vi "Get Description of Shared Variables.vi"(8 "error in":errorcluster, 11 "Variable References In":refnum<k21>[](array[refnum])) -> (0 "error out":errorcluster, 2 "Variable Descriptions":T1[](array[typedef]), 3 "Variable References Out":refnum<k21>[](array[refnum]))   [LabVIEW 2017, in "Shared Variables Library.lvlib"]
doc: "Retrieves the Name, URL and Datatype from an array of shared variable references."
uses:
  Shared Variables Library.lvlib
  Typedefs/Shared Variable Properties--Cluster.ctl
  <resource>/objmgr/ni.var.rc
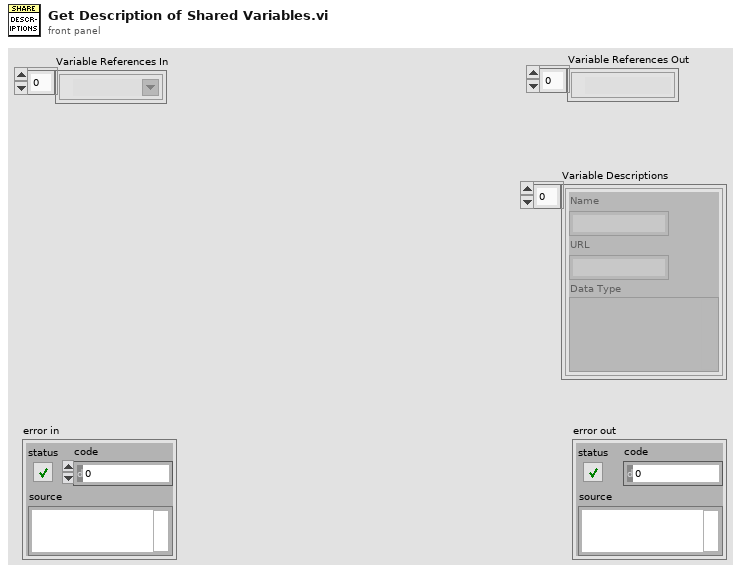
[diagram p1: front panel]
types:
  T1 = typedef "Shared Variables Library.lvlib/Shared Variable Properties--Cluster.ctl" = cluster{"Name":string, "URL":string, "Data Type":variant}
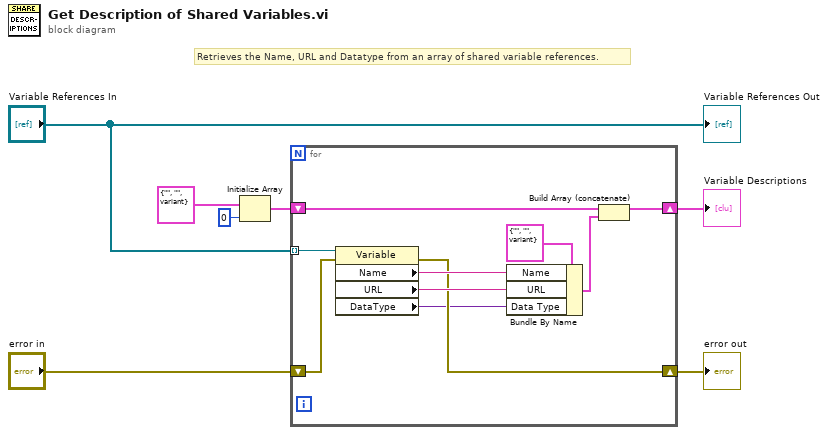
[diagram p0: block diagram]
diagram:
  # "Retrieves the Name, URL and Datatype from an array of shared variable references."
  n1 = Initialize Array(T1 {"Name"="", "URL"="", "Data Type"=variant} ("Shared Variable Data"), 0 ("dimension size")) -> (w4:T1[])
  n2 = for {
    tunnel: "Variable References In" -> [w17] mode=indexing
    shift-right: [w15] -> w5
    shift-left: w4 -> [w16]
    shift-right: [w11] -> w7
    shift-left: "error in" -> [w14]
    n3 = property class="Variable"(reference=w17, error in=w14) -> (error out=w11:errorcluster, "Name"=w13:string, "URL"=w12:string, "DataType"=w10:variant)  [unwired: 1 out]
    n4 = Bundle By Name(cluster=T1 {"Name"="", "URL"="", "Data Type"=variant} ("Shared Variable Data"), "Name"=w13, "URL"=w12, "Data Type"=w10) -> (w8:T1)
    n5 = Build Array (concatenate)(w16, w8) -> (w15:T1[])
  }
  "error out" <- w7
  "Variable Descriptions" <- w5
  "Variable References Out" <- "Variable References In"
